vi "MT_generate_signal6.vi"(7 "Direction":bool, 8 "error in (no error)":errorcluster, 9 "# cycles":dbl, 10 "frequency":dbl, 11 "amplitude":dbl) -> (0 "error out":errorcluster, 2 "signals out":dbl[][](array[numeric]), 3 "# samples":dbl)   [LabVIEW 2019]
uses:
  <vilib>/Analysis/NI_AALBase.lvlib
panel:
  in  "x":dbl=0.3 min=-1.0 max=1.0 step=0.05
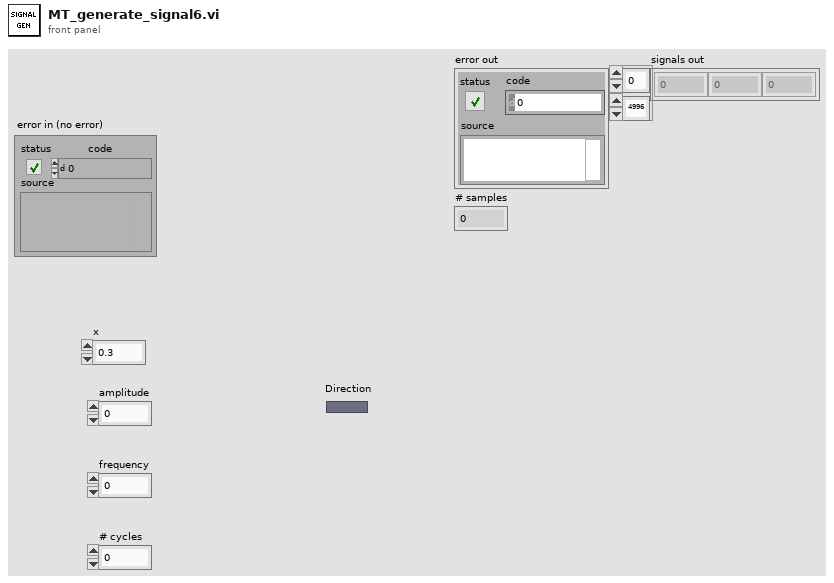
[diagram p1: front panel]
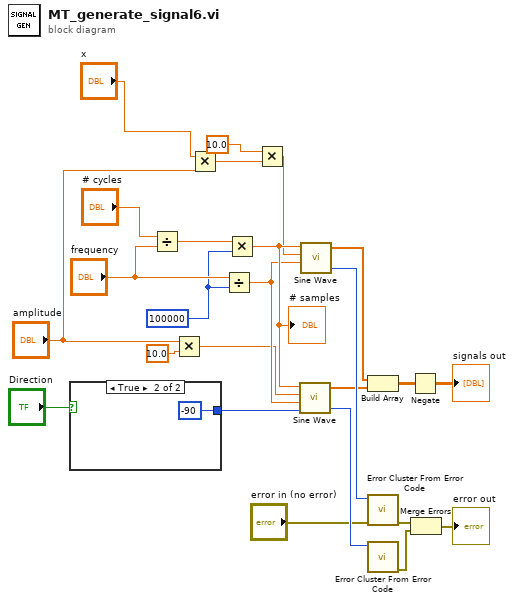
[diagram p0: block diagram]
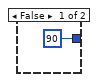
[diagram p2: hidden frame]
diagram:
  w22 = 100000
  n1 = case shown="True" "Direction" {
    tunnel: [90 -90] -> w10
    frame False {
    }
    frame True {
    }
  }
  n2 = Divide(x="# cycles", y="frequency") -> (x/y=w23:dbl)
  n3 = Multiply(x="amplitude", y=10.0) -> (x*y=w18:dbl)
  n4 = Multiply(x="x", y="amplitude") -> (x*y=w3:dbl)
  n5 = Divide(x="frequency", y=w22) -> (x/y=w20:dbl)
  n6 = Multiply(x=w23, y=w22) -> (x*y=w21:dbl)
  "# samples" <- w21
  n7 = Multiply(x=10.0, y=w3) -> (x*y=w2:dbl)
  n8 = call <vilib>:"Sine Wave.vi"("samples"=w21, "amplitude"=w18, "frequency"=w20, "phase in"=w10) -> ("sine wave"=w7:dbl[], "error"=w16:i32)  [unwired: 1 in, 1 out]
  n9 = call <vilib>:"Sine Wave.vi"("samples"=w21, "amplitude"=w2, "frequency"=w20) -> ("sine wave"=w8:dbl[], "error"=w17:i32)  [unwired: 2 in, 1 out]
  n10 = Build Array(w8, w7) -> (w6:dbl[][])
  n11 = call <vilib>:"Error Cluster From Error Code.vi"("error in (no error)"="error in (no error)", "error code (0)"=w17) -> ("error out"=w14:errorcluster)  [unwired: 7 in]
  n12 = call <vilib>:"Error Cluster From Error Code.vi"("error code (0)"=w16) -> ("error out"=w13:errorcluster)  [unwired: 8 in]
  n13 = Negate(x=w6) -> (-x=→"signals out":dbl[][])
  n14 = Merge Errors(w14, w13) -> (→"error out":errorcluster)
